vi "test_ClientFGV_GetClientErrors_ClientNotCreated.vi"(8 "error in":errorcluster) -> (0 "error out":errorcluster, 2 "result":string, 3 "pass":bool)   [LabVIEW 2020, in "MeasurementServerTests.lvlib" / "gRPC Utilities Tests.lvlib"]
uses:
  gRPC Utilities Tests.lvlib
  Runtime/MeasurementLink gRPC Utilities/gRPC Client Pool Helpers/Action.ctl
  Action.ctl
  Runtime/MeasurementLink gRPC Utilities/MeasurementLink gRPC Utilities.lvlib
  MeasurementServerTests.lvlib
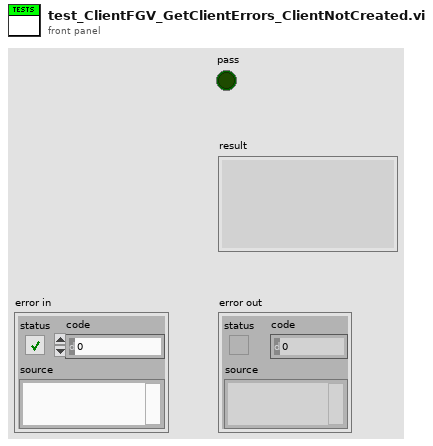
[diagram p1: front panel]
types:
  T1 = typedef "Action.ctl" = enum16{"Increment Id", "Reset", "Error on Next Call"}
  T2 = typedef "MeasurementLink gRPC Utilities.lvlib/Action.ctl" = enum16{"Get Client", "Recreate Client"}
  T3 = typedef "grpc-lvsupport-release.lvlib/grpcId.ctl" = u64
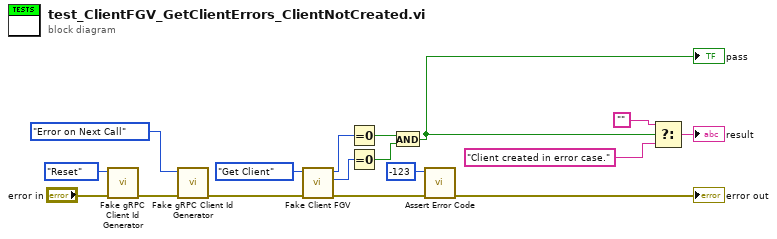
[diagram p0: block diagram]
diagram:
  n1 = call "Fake gRPC Client Id Generator.vi"("error in"="error in", "action"=Action."Reset") -> ("error out"=w9:errorcluster)  [unwired: 8 in, 1 out]
  n2 = call "Fake gRPC Client Id Generator.vi"("error in"=w9, "action"=Action."Error on Next Call") -> ("error out"=w10:errorcluster)  [unwired: 8 in, 1 out]
  n3 = call "Fake Client FGV.vi"("error in"=w10, "action"=Action."Get Client") -> ("error out"=w3:errorcluster, "unique id out"=w7:u64, "grpc client id"=w8:T3)  [unwired: 7 in]
  n4 = Equal To 0?(x=w8) -> (x = 0?=w6:bool)
  n5 = Equal To 0?(x=w7) -> (x = 0?=w5:bool)
  n6 = And(x=w6, y=w5) -> (x .and. y?=w4:bool)
  "pass" <- w4
  n7 = call "Assert Error Code.vi"("error in"=w3, "expected error code"=-123) -> ("error out"=→"error out":errorcluster)  [unwired: 7 in, 2 out]
  n8 = Select(t="", s=w4, f="Client created in error case.") -> (s? t:f=→"result":string)
